vi "readSVs.vi"(8 "error in (no error)":errorcluster, 11 "ApplicationHandler in":refnum<class "ApplicationHandler.lvclass">) -> (0 "error out":errorcluster, 3 "ApplicationHandler out":refnum<class "ApplicationHandler.lvclass">)   [LabVIEW 2013, in "ComponentData.lvlib" / "ApplicationHandler.lvclass"]
uses:
  <userlib>/Common/Component/Application/RT/ComponentData/ApplicationHandler/ApplicationHandler.lvclass
  <userlib>/Common/Component/Application/RT/ComponentData/ApplicationHandler/ApplicationHandler.lvclass/ApplicationHandler.ctl
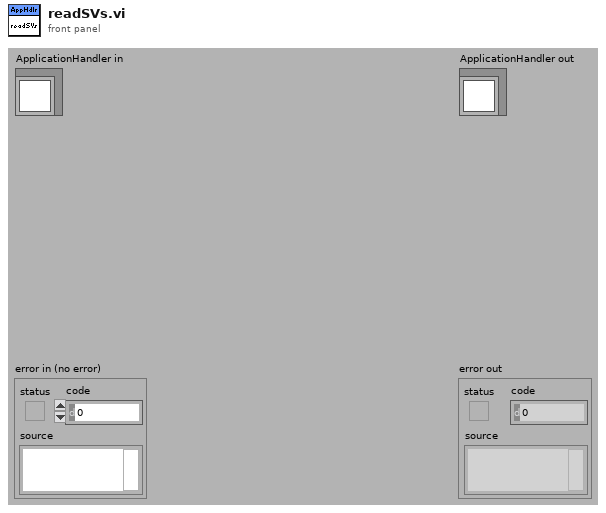
[diagram p1: front panel]
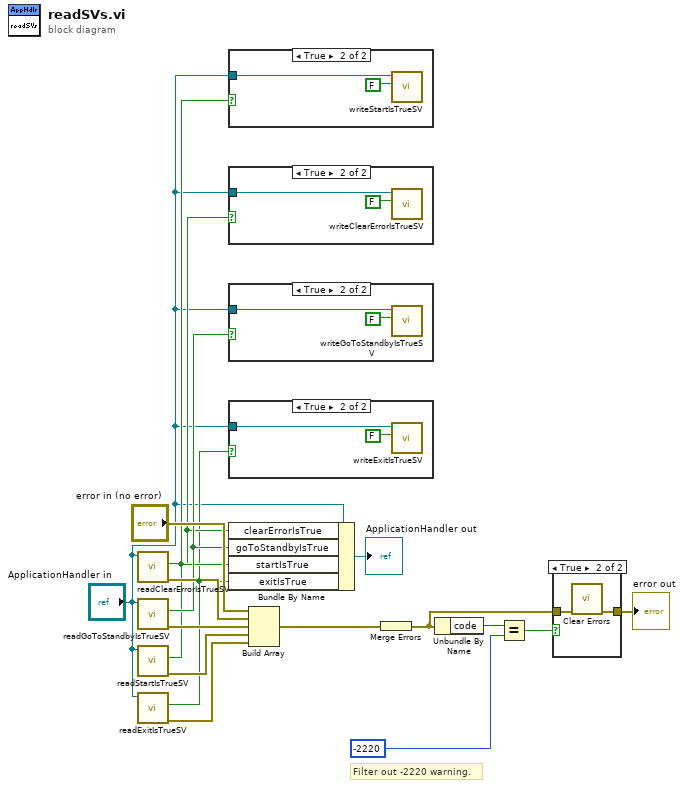
[diagram p0: block diagram]
diagram:
  # "Filter out -2220 warning."
  n1 = call-dynamic "readClearErrorIsTrueSV.vi"("ApplicationHandler in"="ApplicationHandler in") -> ("error out"=w11:errorcluster, "ClearErrorIsTrue"=w3:bool)  [unwired: 8 in, 1 out]
  n2 = call-dynamic "readGoToStandbyIsTrueSV.vi"("ApplicationHandler in"="ApplicationHandler in") -> ("error out"=w10:errorcluster, "goToStandbyIsTrue"=w5:bool)  [unwired: 8 in, 1 out]
  n3 = call-dynamic "readStartIsTrueSV.vi"("ApplicationHandler in"="ApplicationHandler in") -> ("error out"=w7:errorcluster, "startIsTrue"=w4:bool)  [unwired: 8 in, 1 out]
  n4 = call-dynamic "readExitIsTrueSV.vi"("ApplicationHandler in"="ApplicationHandler in") -> ("error out"=w6:errorcluster, "exitIsTrue"=w2:bool)  [unwired: 8 in, 1 out]
  n5 = case shown="True" w4 {
    tunnel: "ApplicationHandler in" -> [_ w18]
    frame False {
    }
    frame True {
      n6 = call-dynamic "writeStartIsTrueSV.vi"("startIsTrue"=FALSE, "ApplicationHandler in"=w18) -> ()  [unwired: 8 in, 2 out]
    }
  }
  n7 = case shown="True" w3 {
    tunnel: "ApplicationHandler in" -> [_ w20]
    frame False {
    }
    frame True {
      n8 = call-dynamic "writeClearErrorIsTrueSV.vi"("clearErrorIsTrue"=FALSE, "ApplicationHandler in"=w20) -> ()  [unwired: 8 in, 2 out]
    }
  }
  n9 = case shown="True" w5 {
    tunnel: "ApplicationHandler in" -> [_ w23]
    frame False {
    }
    frame True {
      n10 = call-dynamic "writeGoToStandbyIsTrueSV.vi"("goToStandbyIsTrue"=FALSE, "ApplicationHandler in"=w23) -> ()  [unwired: 8 in, 2 out]
    }
  }
  n11 = case shown="True" w2 {
    tunnel: "ApplicationHandler in" -> [_ w24]
    frame False {
    }
    frame True {
      n12 = call-dynamic "writeExitIsTrueSV.vi"("exitIsTrue"=FALSE, "ApplicationHandler in"=w24) -> ()  [unwired: 8 in, 2 out]
    }
  }
  n13 = Bundle By Name(cluster="ApplicationHandler in", "clearErrorIsTrue"=w3, "goToStandbyIsTrue"=w5, "startIsTrue"=w4, "exitIsTrue"=w2) -> (→"ApplicationHandler out":refnum<class "ApplicationHandler.lvclass">)
  n14 = Build Array("error in (no error)", w11, w10, w7, w6) -> (w17:errorcluster[])
  n15 = Merge Errors(w17) -> (w13:errorcluster)
  n16 = Unbundle By Name(w13) -> ("code"=w16:i32)
  n17 = Equal?(x=w16, y=-2220) -> (x = y?=w14:bool)
  n18 = case shown="True" w14 {
    tunnel: w13 -> [w26 w28]
    tunnel: [w26 w27] -> w8
    frame False {
    }
    frame True {
      n19 = call <vilib>:"Clear Errors.vi"("error in (no error)"=w28) -> ("error out"=w27:errorcluster)  [unwired: 6 in]
    }
  }
  "error out" <- w8
